vi "GeneratePoint Z CV Approach.vi"(11 "Input":T2) -> (0 "output cluster":T1)   [LabVIEW 2023]
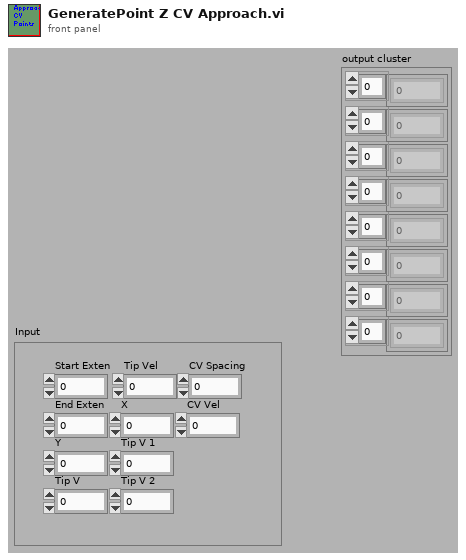
[diagram p1: front panel]
types:
  T1 = cluster{dbl[], dbl[], dbl[], dbl[], dbl[], dbl[], dbl[], dbl[]}
  T2 = cluster{"Start Exten":dbl, "End Exten":dbl, "Tip Vel":dbl, "X":dbl, "Y":dbl, "Tip V":dbl, "Tip V 1":dbl, "Tip V 2":dbl, "CV Spacing":dbl, "CV Vel":dbl}
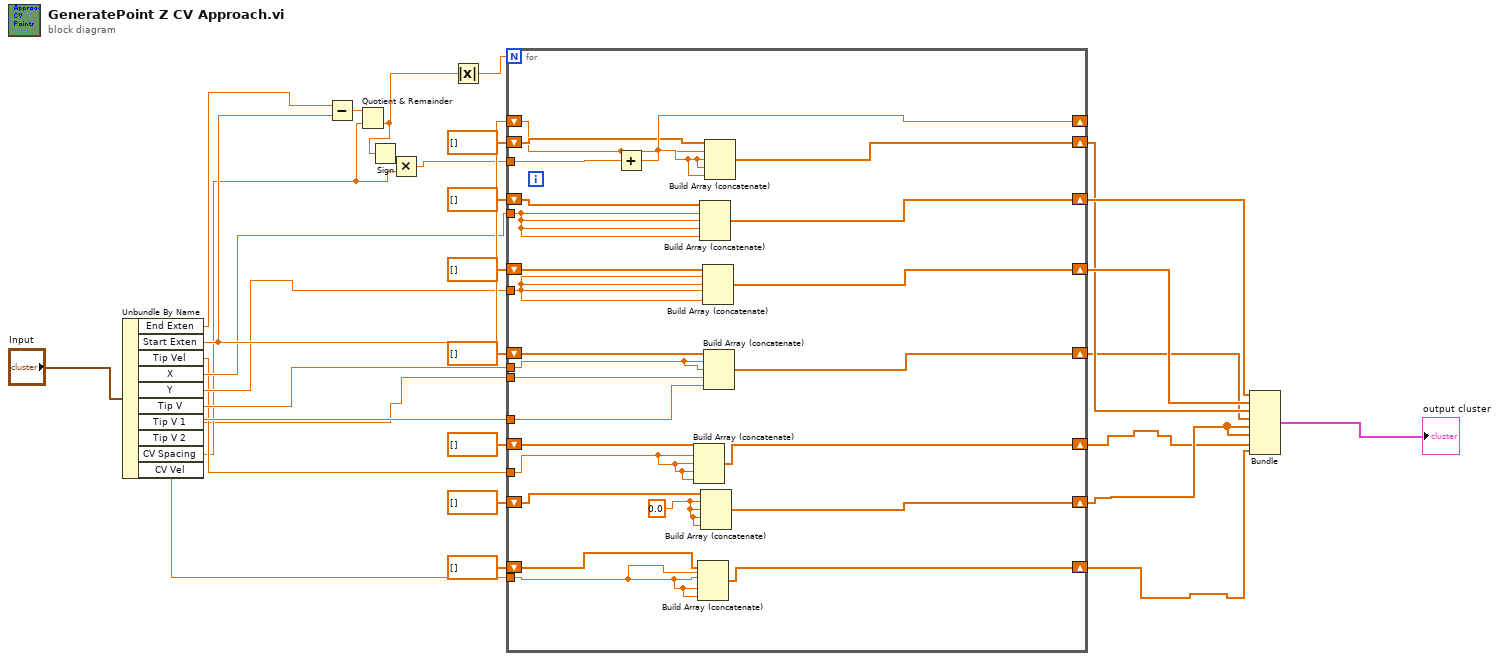
[diagram p0: block diagram]
diagram:
  n1 = Unbundle By Name("Input") -> ("End Exten"=w29:dbl, "Start Exten"=w28:dbl, "Tip Vel"=w23:dbl, "X"=w27:dbl, "Y"=w26:dbl, "Tip V"=w25:dbl, "Tip V 1"=w1:dbl, "Tip V 2"=w24:dbl, "CV Spacing"=w13:dbl, "CV Vel"=w22:dbl)
  n2 = Subtract(x=w29, y=w28) -> (x-y=w31:dbl)
  n3 = Quotient & Remainder(x=w31, y=w13) -> (floor(x/y)=w15:dbl)  [unwired: 1 out]
  n4 = Sign(1:w15) -> (0:w14:dbl)
  n5 = Multiply(x=w14, y=w13) -> (x*y=w12:dbl)
  n6 = Absolute Value(x=w15) -> (abs(x)=w16:dbl)
  n7 = for {
    N: w16 -> [_]
    shift-right: [w55] -> _
    shift-left: w28 -> [w34]
    tunnel: w12 -> [w36]
    tunnel: w27 -> [w54]
    tunnel: w26 -> [w52]
    tunnel: w25 -> [w48]
    tunnel: w1 -> [w50]
    tunnel: w24 -> [w49]
    tunnel: w23 -> [w33]
    tunnel: w22 -> [w32]
    shift-right: [w56] -> w19
    shift-left: dbl[] [] -> [w43]
    shift-right: [w53] -> w21
    shift-left: dbl[] [] -> [w42]
    shift-right: [w51] -> w20
    shift-left: dbl[] [] -> [w41]
    shift-right: [w47] -> w18
    shift-left: dbl[] [] -> [w40]
    shift-right: [w46] -> w2
    shift-left: dbl[] [] -> [w39]
    shift-right: [w45] -> w3
    shift-left: dbl[] [] -> [w38]
    shift-right: [w44] -> w4
    shift-left: dbl[] [] -> [w37]
    w35 = 0.0
    n8 = Add(x=w34, y=w36) -> (x+y=w55:dbl)
    n9 = Build Array (concatenate)(w39, w33, w33, w33, w33) -> (w46:dbl[])
    n10 = Build Array (concatenate)(w37, w32, w32, w32, w32) -> (w44:dbl[])
    n11 = Build Array (concatenate)(w42, w54, w54, w54, w54) -> (w53:dbl[])
    n12 = Build Array (concatenate)(w38, w35, w35, w35, w35) -> (w45:dbl[])
    n13 = Build Array (concatenate)(w41, w52, w52, w52, w52) -> (w51:dbl[])
    n14 = Build Array (concatenate)(w40, w48, w48, w50, w49) -> (w47:dbl[])
    n15 = Build Array (concatenate)(w43, w34, w55, w55, w55) -> (w56:dbl[])
  }
  n16 = Bundle(w21, w20, w19, w18, w3, w3, w2, w4) -> (→"output cluster":T1)  [unwired: 1 in]
